vi "XY Graph Update New Plot Name.vi"(6 "Plot Created?":bool, 8 "error in (no error)":errorcluster, 9 "Actual Plot ID":i32, 10 "New Plot Name":string, 11 "XYGraph in":refnum<vi>) -> (0 "error out":errorcluster)   [LabVIEW 2021, in "XY Graph Add-Ons.lvlib"]
uses:
  XY Graph Add-Ons.lvlib
  Strings/Strings.lvlib
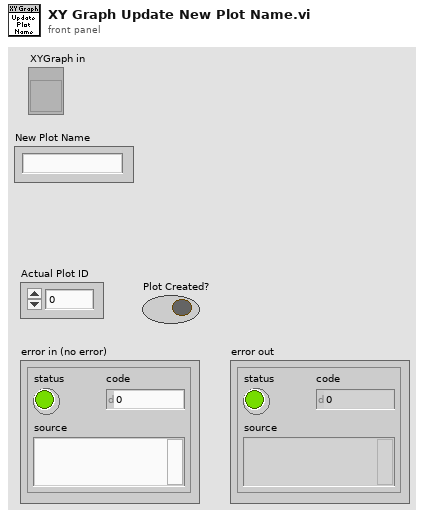
[diagram p1: front panel]
types:
  T1 = typedef "XY Graph Add-Ons.lvlib/XY Graph Refnum.ctl" = refnum<vi>
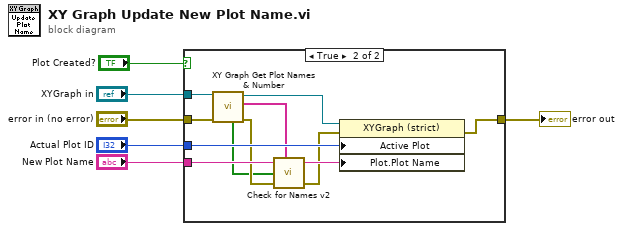
[diagram p0: block diagram]
diagram:
  n1 = case shown="True" "Plot Created?" {
    tunnel: "XYGraph in" -> [_ w16]
    tunnel: "error in (no error)" -> [w7 w14]
    tunnel: [w7 w18] -> w4
    tunnel: "Actual Plot ID" -> [_ w17]
    tunnel: "New Plot Name" -> [_ w13]
    frame False {
    }
    frame True {
      n2 = call "XY Graph Get Plot Names & Number.vi"("error in (no error)"=w14, "XYGraph in"=w16) -> ("error out"=w12:errorcluster, "Plot Names"=w11:string[], "XYGraph out"=w15:T1, "Empty Plots?"=w8:bool[])  [unwired: 4 in, 2 out]
      n3 = call "Check for Names v2.vi"("New Name"=w13, "Name List"=w11, "Empty Plots?"=w8, "Error In"=w12) -> ("New Name"=w10:string, "Error Out"=w9:errorcluster)  [unwired: 2 in, 2 out]
      n4 = property class="XYGraph (strict)"(reference=w15, error in=w9, "Active Plot"=w17, "Plot.Plot Name"=w10) -> (error out=w18:errorcluster)  [unwired: 1 out]
    }
  }
  "error out" <- w4
